vi "Main.vi"() -> ()   [LabVIEW 2017]
uses:
  <vilib>/userdefined/High Color/IMAQdx.ctl
  <vilib>/ErrorRing/Error Ring.xnode
  <vilib>/vision/driver/NI_Vision_Acquisition_Software.lvlib
panel:
  out "Images saved in:":path
  in  "Prefix Filename":string="GGS-Image-"
  in  "milliseconds to wait":u32=5000
  out "Taking Picture":bool
  out "Ready":bool
  in  "Take Pictures":bool
  in  "Image Quality":u32=750 max=1000 step=10
  in  "stop":bool
  out "USB Camera Image":T1(plugin-control)
  in  "Session In":T2
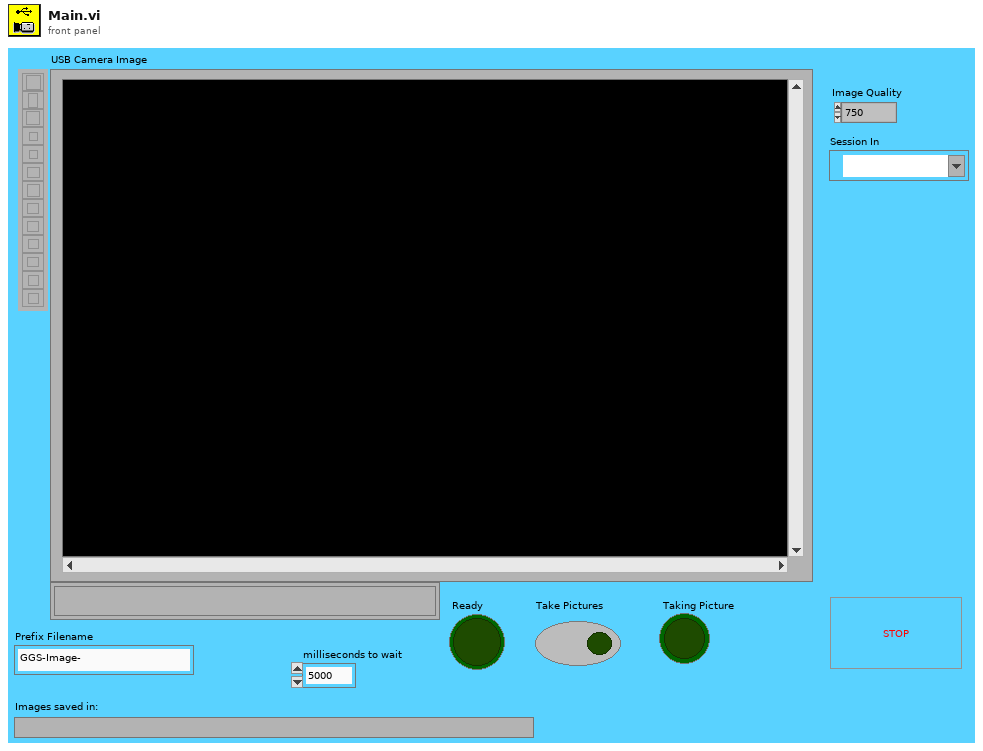
[diagram p1: front panel]
types:
  T1 = typedef "IMAQ Image.ctl" = refnum<image>
  T2 = typedef "IMAQdx.ctl" = refnum<k21>
  T3 = typedef "Image Type" = u32
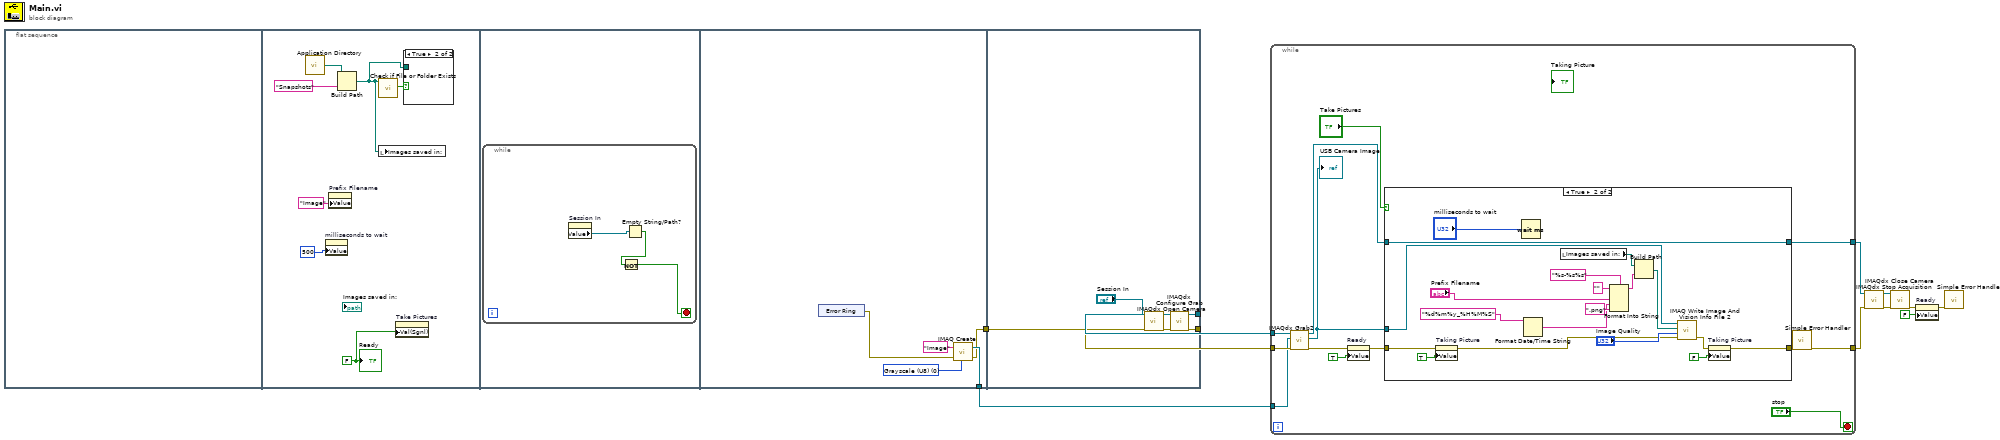
[diagram p0: block diagram]
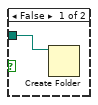
[diagram p2: hidden frame]
diagram:
  n1 = flat-sequence {
    tunnel: [w26] -> w9
    tunnel: [w23] -> w4
    tunnel: [w33] -> w11
    tunnel: [w31] -> w10
    tunnel: w4 -> [w29]
    frame #0 {
    }
    frame #1 {
      w12 = FALSE ("Take Pictures")
      n2 = call <vilib>:"Application Directory.vi"() -> ("Application Directory"=w18:path)
      n3 = property on="milliseconds to wait" class="DigNum (strict)"("Value"=u32 500 ("milliseconds to wait")) -> ()  [unwired: 2 in, 2 out]
      n4 = property on="Prefix Filename" class="Str"("Value"="Image" ("Prefix Filename")) -> ()  [unwired: 2 in, 2 out]
      n5 = Build Path(base path=w18, name or relative path="Snapshots") -> (appended path=w14:path)
      n6 = call <vilib>:"Check if File or Folder Exists.vi"("path"=w14) -> ("file or folder exists?"=w17:bool)  [unwired: 8 in, 2 out]
      n7 = local write "Images saved in:"(w14) -> ()
      n8 = property on="Take Pictures" class="Bool (strict)"("Val(Sgnl)"=w12) -> ()  [unwired: 2 in, 2 out]
      n9 = case shown="True" w17 {
        tunnel: w14 -> [w19 _]
        frame False {
          n10 = Create Folder(path (use dialog)=w19) -> ()  [unwired: 2 in, 3 out]
        }
        frame True {
        }
      }
      "Ready" <- w12
    }
    frame #2 {
      n11 = while {
        stop <- w20 stop-if-true
        n12 = property on="Session In" class="IMAQdx (strict)"() -> ("Value"=w22:T2)  [unwired: 2 in, 2 out]
        n13 = Empty String/Path?(string/path=w22) -> (empty?=w21:bool)
        n14 = Not(x=w21) -> (.not. x?=w20:bool)
      }
    }
    frame #3 {
      w27 = T3 0 items=["Grayscale (U8)", "Grayscale (I16)", "Grayscale (SGL)", "Complex (CSG)", "RGB (U32)", "HSL (U32)", "RGB (U64)", "Grayscale (U16)"] ("Image Type")
      n15 = xnode "Error Ring"() -> ("error out"=w24:errorcluster)
      n16 = call "IMAQ Create"("Image Name"="Image", "Image Type"=w27, "error in (no error)"=w24) -> ("New Image"=w26:T1, "error out"=w23:errorcluster)  [unwired: 2 in]
    }
    frame #4 {
      n17 = call <vilib>:"IMAQdx Open Camera.vi"("error in"=w29, "Session In"="Session In") -> ("error out"=w32:errorcluster, "Session Out"=w34:T2)  [unwired: 8 in]
      n18 = call <vilib>:"IMAQdx Configure Grab.vi"("error in"=w32, "Session In"=w34) -> ("error out"=w31:errorcluster, "Session Out"=w33:T2)  [unwired: 8 in]
    }
  }
  n19 = while {
    tunnel: w11 -> [w47]
    tunnel: w10 -> [w46]
    tunnel: w9 -> [w41]
    tunnel: [w36] -> w8
    tunnel: [w35] -> w7
    stop <- "stop" stop-if-true
    n20 = call <vilib>:"IMAQdx Grab2.vi"("error in"=w46, "Image In"=w41, "Session In"=w47) -> ("error out"=w39:errorcluster, "Image Out"=w43:T1, "Session Out"=w37:T2)  [unwired: 5 in, 1 out]
    "USB Camera Image" <- w43
    n21 = property on="Ready" class="Bool (strict)"(error in=w39, "Value"=TRUE ("Ready")) -> (error out=w38:errorcluster)  [unwired: 1 in, 1 out]
    n22 = case shown="True" "Take Pictures" {
      tunnel: w38 -> [w49 w67]
      tunnel: w43 -> [_ w61]
      tunnel: [w49 w64] -> w42
      tunnel: w37 -> [w48 w60]
      tunnel: [w48 w60] -> w35
      frame False {
      }
      frame True {
        n23 = property on="Taking Picture" class="Bool (strict)"(error in=w67, "Value"=TRUE ("Taking Picture")) -> (error out=w62:errorcluster)  [unwired: 1 in, 1 out]
        n24 = Wait (ms)(milliseconds to wait="milliseconds to wait") -> ()  [unwired: 1 out]
        n25 = Format Date/Time String(time format string (%c)="%d%m%y_%H%M%S") -> (date/time string=w51:string)  [unwired: 2 in]
        n26 = local read "Images saved in:"() -> (w50:path)
        n27 = Format Into String(format string="%s-%s%s", initial string="", "Prefix Filename", w51, ".png" ("input 3")) -> (resulting string=w54:string)  [unwired: 1 in, 1 out]
        n28 = Build Path(base path=w50, name or relative path=w54) -> (appended path=w53:path)
        n29 = call "IMAQ Write Image And Vision Info File 2"("error in (no error)"=w62, "Image Quality"="Image Quality", "File Path"=w53, "Image"=w61) -> ("error out"=w63:errorcluster)  [unwired: 6 in, 1 out]
        n30 = property on="Taking Picture" class="Bool (strict)"(error in=w63, "Value"=FALSE ("Taking Picture")) -> (error out=w64:errorcluster)  [unwired: 1 in, 1 out]
      }
    }
    n31 = call <vilib>:"Simple Error Handler.vi"("error in (no error)"=w42) -> ("error out"=w36:errorcluster)  [unwired: 4 in, 4 out]
  }
  n32 = call <vilib>:"IMAQdx Stop Acquisition.vi"("error in"=w8, "Session In"=w7) -> ("error out"=w6:errorcluster, "Session Out"=w5:T2)  [unwired: 8 in]
  n33 = call <vilib>:"IMAQdx Close Camera.vi"("error in"=w6, "Session In"=w5) -> ("error out"=w3:errorcluster)  [unwired: 9 in]
  n34 = property on="Ready" class="Bool (strict)"(error in=w3, "Value"=FALSE ("Ready")) -> (error out=w2:errorcluster)  [unwired: 1 in, 1 out]
  n35 = call <vilib>:"Simple Error Handler.vi"("error in (no error)"=w2) -> ()  [unwired: 4 in, 5 out]
